vi "WIDTH_DIV_2.vi"() -> (0 "WIDTH_DIV_2":i16=200)   [LabVIEW 2020]
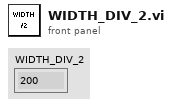
[diagram p1: front panel]
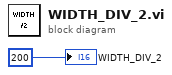
[diagram p0: block diagram]
diagram:
  "WIDTH_DIV_2" <- i16 200
